vi "실습 1-4.vi"() -> ()   [LabVIEW 2014]
panel:
  in  "Run":bool
  in  "정지":bool
  out "웨이브폼 차트":dbl(graph)
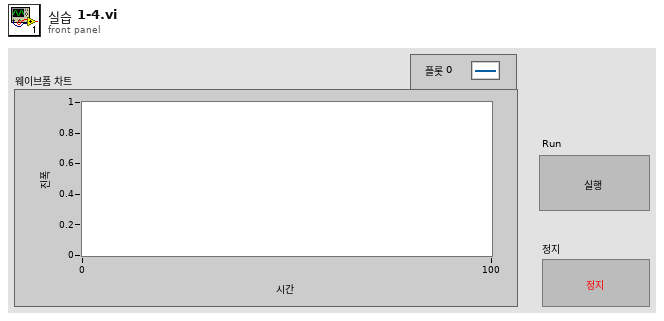
[diagram p1: front panel]
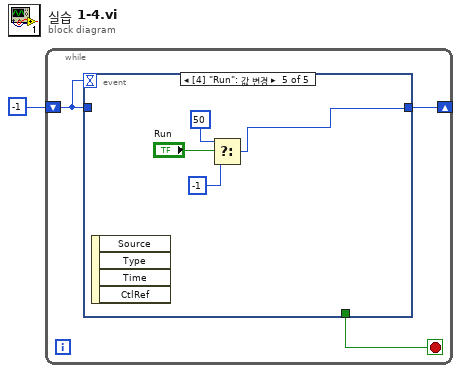
[diagram p0: block diagram]
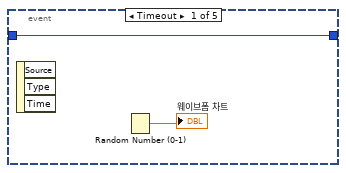
[diagram p2: hidden frame]
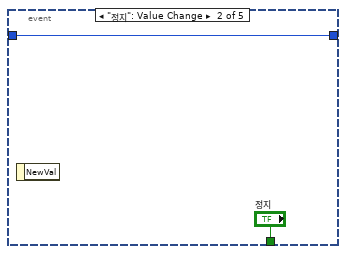
[diagram p3: hidden frame]
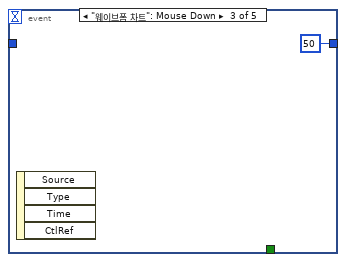
[diagram p4: hidden frame]
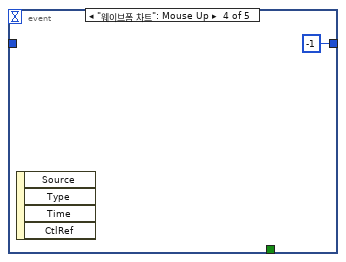
[diagram p5: hidden frame]
diagram:
  n1 = while {
    shift-right: [w2] -> _
    shift-left: -1 -> [w3]
    stop <- w4 stop-if-true
    n2 = event shown="[4] \"Run\": 값 변경" {
      selector: _ -> [_ _ _ _ _]
      dyn-events: _ -> [_ _ _ _ _]
      timeout: w3 -> [_ _ _ _ _]
      tunnel: [_ "정지" _ _ _] -> w4
      tunnel: w3 -> [w5 w7 _ _ _]
      tunnel: [w5 w7 50 -1 w11] -> w2
      event Timeout {
        n3 = event-data() -> ()  [unwired: 1 in, 3 out]
        n4 = Random Number (0-1)() -> (number: 0 to 1=→"웨이브폼 차트":dbl)
      }
      event "정지": Value Change {
        n5 = event-data() -> ()  [unwired: 1 in, 1 out]
      }
      event "웨이브폼 차트": Mouse Down {
        n6 = event-data() -> ()  [unwired: 1 in, 4 out]
      }
      event "웨이브폼 차트": Mouse Up {
        n7 = event-data() -> ()  [unwired: 1 in, 4 out]
      }
      event "Run": Value Change {
        n8 = event-data() -> ()  [unwired: 1 in, 4 out]
        n9 = Select(t=50, s="Run", f=-1) -> (s? t:f=w11:i32)
      }
    }
  }
